vi "OceanOptics_TriggerPlayground.vi"() -> ()   [LabVIEW 2016]
uses:
  Maya2000 Typedefs/Maya2000 basic info.ctl
  <vilib>/Platform/TimedLoop/XDataNode/timing_clust.ctl
  <vilib>/Platform/TimedLoop/XDataNode/nitl_modes.ctl
  <vilib>/Platform/TimedLoop/XDataNode/wakeup.ctl
  C:/Program Files/Ocean Optics/OmniDriver/OOI_HOME/NETOmniDriver-NET40.dll
  Program Files/Ocean Optics/OmniDriver/OOI_HOME/NETOmniDriver-NET40.dll
  <vilib>/platform/TimedLoop/XDataNode/XDataNode.xnode
  <vilib>/Platform/TimedLoop/XDataNode/XDNodeRunTimeDep.lvlib
panel:
  out "getBufferCapacity 3":i32
  out "isEnableBuffer 2":i16
  out "getExternalTriggerDelayIncrement":i32
  out "read":bool
  out "getBufferCapacity":i32
  out "getNumberOfElements":i32
  out "status":bool
  out "error out":errorcluster
  out "this maya":T1={"This instruments index"=0, "Name+SerialNumber"="MayaPro2000:MAYP111403", "Number Dark pixels"=8, "NumberOfPixels\nper spectrum"=2068, "NumberOf Maya2000 instrm."=2, "MaximumIntegrationTime\n[us]"=1600000000, "MinimumIntegrationTime\n[us]"=7200}
  in  "number of scans to average":i32=1 min=1 step=1
  out "spectrum":cluster{"Y":dbl[], "Y":dbl[]}[](graph)
  in  "stop":bool
  in  "integration time [us]":i32=100000
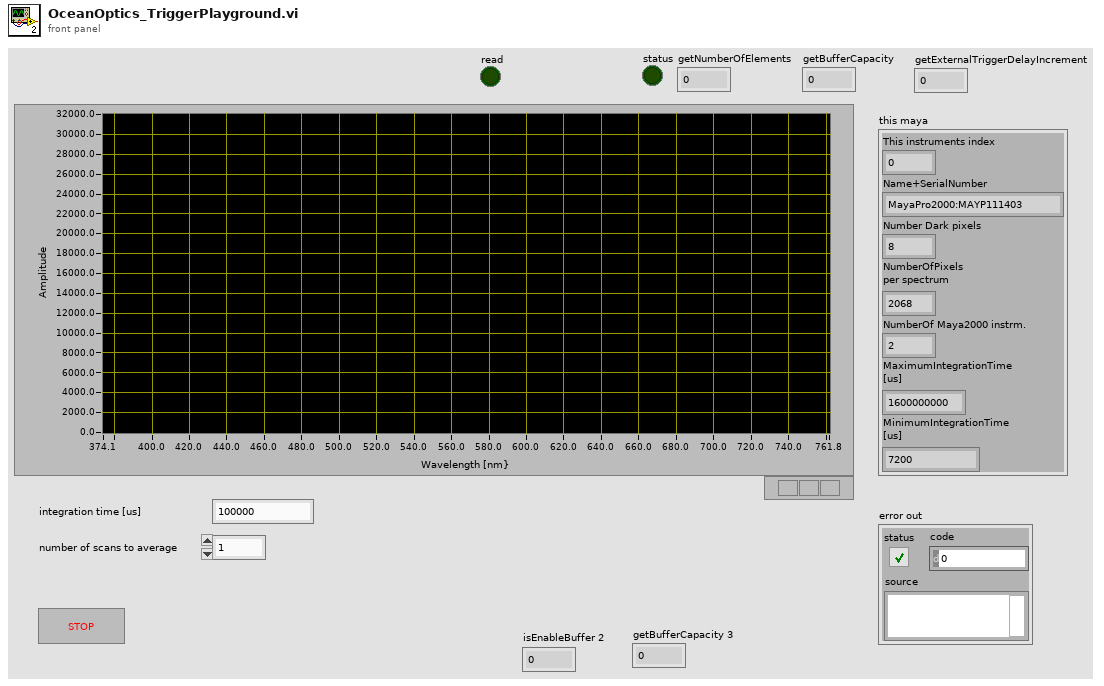
[diagram p1: front panel]
types:
  T1 = typedef "Maya2000 basic info.ctl" = cluster{"This instruments index":i32, "Name+SerialNumber":string, "Number Dark pixels":i32, "NumberOfPixels\nper spectrum":i32, "NumberOf Maya2000 instrm.":i32, "MaximumIntegrationTime\n[us]":i32, "MinimumIntegrationTime\n[us]":i32}
  T2 = typedef "XDNodeRunTimeDep.lvlib/timing_clust.ctl" = cluster{"Expected End [f-1]":u64, "Actual End [f-1]":u64, "Finished Late? [f-1]":bool, "Expected End [i-1]":u64, "Actual End [i-1]":u64, "Finished Late? [i-1]":bool, "Expected Start [i]":u64, "Actual Start [i]":u64, "Expected Start [f]":u64, "Actual Start [f]":u64, "Source Name":string, "Structure Name":string, "Period":i64, "Deadline":i64, "Offset":i64, "Start":i64, "Priority":i32, "Timeout":i32, "Mode":T3, "Wakeup Reason":T4, "Error":errorcluster, "Source Type":string, "Secondary Source Type":string, "Global End Time":u64, "Global Start Time":u64, "Frame Duration":u64, "Iteration Duration":u64, "Assigned CPU":i32, "I/O Scan Engine Mode":u32}
  T3 = typedef "XDNodeRunTimeDep.lvlib/nitl_modes.ctl" = enum32{"No Change", "Process missed periods, maintain original phase", "Discard missed periods, maintain original phase", "Process missed periods, ignore original phase", "Discard missed periods, ignore original phase"}
  T4 = typedef "XDNodeRunTimeDep.lvlib/wakeup.ctl" = enum32{"Normal", "Aborted", "Asynchronous wakeup", "Timing source error", "Timed loop error", "Timeout"}
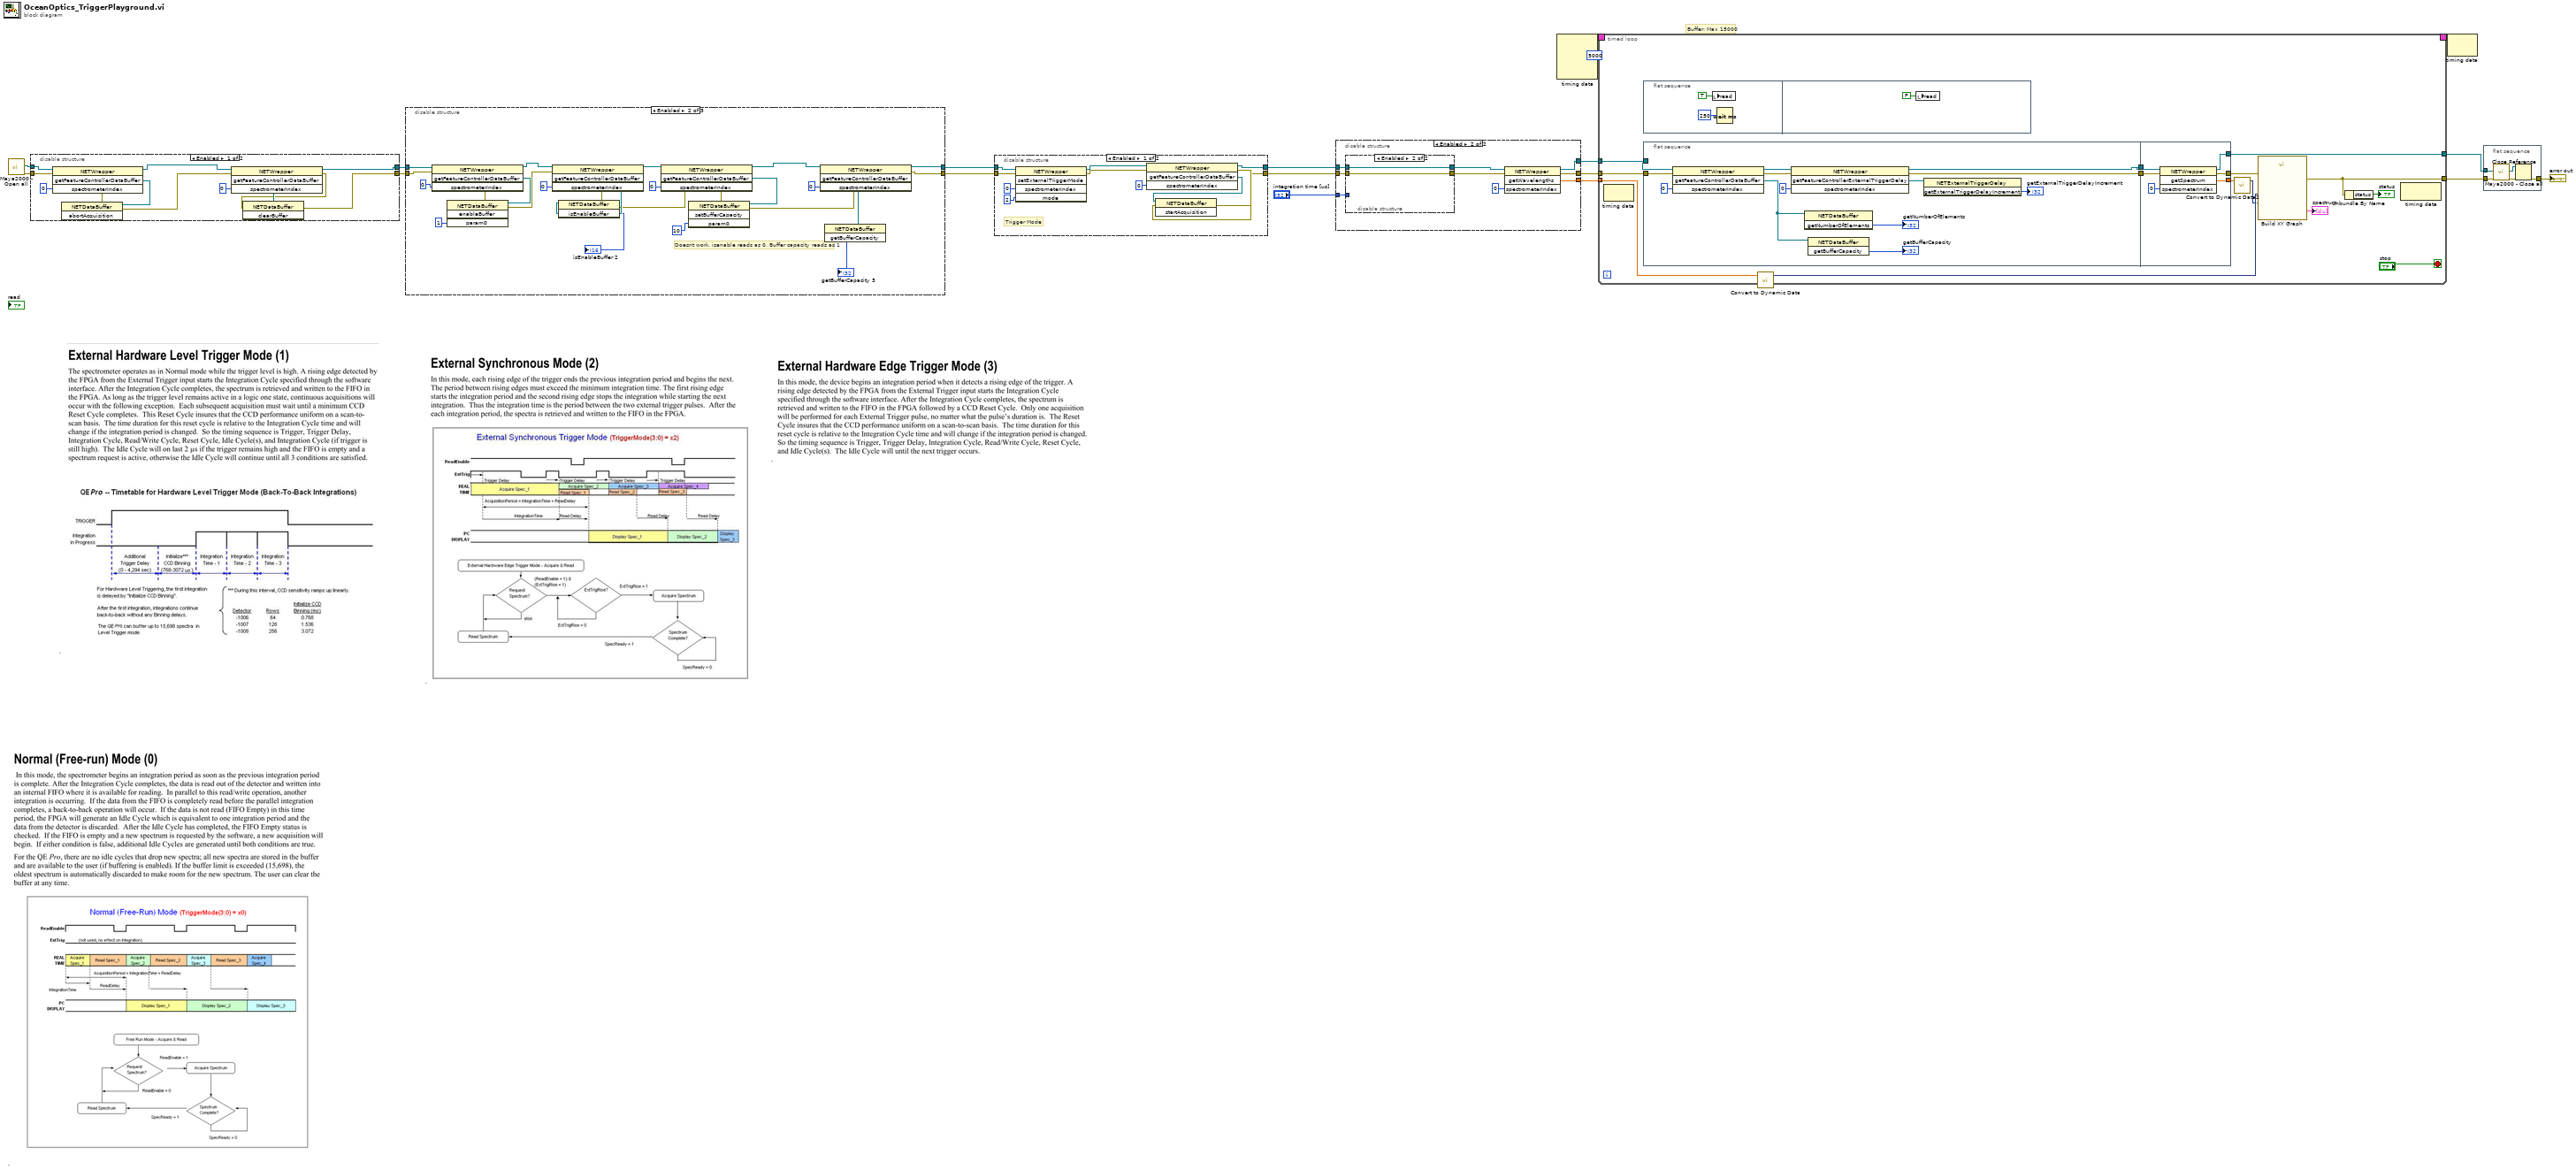
[diagram p0: block diagram]
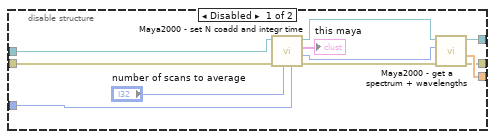
[diagram p6: hidden frame]
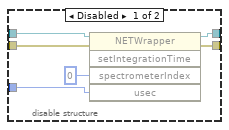
[diagram p7: hidden frame]
diagram:
  # "Buffer: Max 15000"
  n1 = call "Maya2000 - Open all.vi"() -> ("error out"=w14:errorcluster, ".NET Refnum out"=w13:refnum<k24>)  [unwired: 9 in, 1 out]
  n2 = disable-structure shown="Enabled" {
    disable-tunnel: w14 -> [w30 w31]
    disable-tunnel: w13 -> [w29 w32]
    disable-tunnel: [w19 _] -> w6
    disable-tunnel: [w21 _] -> w5
    frame Enabled {
      n3 = invoke class="NETWrapper" method="getFeatureControllerDataBuffer"(reference=w29, error in=w30, "spectrometerIndex"=0) -> (reference out=w25:refnum<k24>, error out=w27:errorcluster, "getFeatureControllerDataBuffer"=w28:refnum<k24>)  [unwired: 1 in, 1 out]
      n4 = invoke class="NETDataBuffer" method="abortAcquisition"(reference=w28, error in=w27) -> (error out=w22:errorcluster)  [unwired: 1 in, 2 out]
      n5 = invoke class="NETWrapper" method="getFeatureControllerDataBuffer"(reference=w25, error in=w22, "spectrometerIndex"=0) -> (reference out=w21:refnum<k24>, error out=w20:errorcluster, "getFeatureControllerDataBuffer"=w23:refnum<k24>)  [unwired: 1 in, 1 out]
      n6 = invoke class="NETDataBuffer" method="clearBuffer"(reference=w23, error in=w20) -> (error out=w19:errorcluster)  [unwired: 1 in, 2 out]
    }
    frame Disabled {
    }
  }
  n7 = disable-structure shown="Enabled" {
    disable-tunnel: w6 -> [_ w41 _]
    disable-tunnel: w5 -> [_ w42 _]
    disable-tunnel: [_ w46 _] -> w4
    disable-tunnel: [_ w45 _] -> w3
    frame Disabled {
    }
    frame Enabled {
      # "Doesnt work, isenable reads as 0, Buffer capacity reads as 1"
      n8 = invoke class="NETWrapper" method="getFeatureControllerDataBuffer"(reference=w42, error in=w41, "spectrometerIndex"=0) -> (reference out=w43:refnum<k24>, error out=w40:errorcluster, "getFeatureControllerDataBuffer"=w39:refnum<k24>)  [unwired: 1 in, 1 out]
      n9 = invoke class="NETDataBuffer" method="enableBuffer"(reference=w39, error in=w40, "param0"=i16 1) -> (error out=w38:errorcluster)  [unwired: 1 in, 3 out]
      n10 = invoke class="NETWrapper" method="getFeatureControllerDataBuffer"(reference=w43, error in=w38, "spectrometerIndex"=0) -> (reference out=w49:refnum<k24>, error out=w37:errorcluster, "getFeatureControllerDataBuffer"=w48:refnum<k24>)  [unwired: 1 in, 1 out]
      n11 = invoke class="NETDataBuffer" method="isEnableBuffer"(reference=w48, error in=w37) -> (error out=w36:errorcluster, "isEnableBuffer"=→"isEnableBuffer 2":i16)  [unwired: 1 in, 1 out]
      n12 = invoke class="NETWrapper" method="getFeatureControllerDataBuffer"(reference=w49, error in=w36, "spectrometerIndex"=0) -> (reference out=w54:refnum<k24>, error out=w35:errorcluster, "getFeatureControllerDataBuffer"=w56:refnum<k24>)  [unwired: 1 in, 1 out]
      n13 = invoke class="NETDataBuffer" method="setBufferCapacity"(reference=w56, error in=w35, "param0"=10) -> (error out=w34:errorcluster)  [unwired: 1 in, 3 out]
      n14 = invoke class="NETWrapper" method="getFeatureControllerDataBuffer"(reference=w54, error in=w34, "spectrometerIndex"=0) -> (reference out=w46:refnum<k24>, error out=w45:errorcluster, "getFeatureControllerDataBuffer"=w55:refnum<k24>)  [unwired: 1 in, 1 out]
      n15 = invoke class="NETDataBuffer" method="getBufferCapacity"(reference=w55) -> ("getBufferCapacity"=→"getBufferCapacity 3":i32)  [unwired: 2 in, 2 out]
    }
    frame Disabled {
    }
  }
  n16 = disable-structure shown="Enabled" {
    disable-tunnel: [w58 w69] -> w1
    disable-tunnel: [w60 w70] -> w2
    disable-tunnel: w4 -> [w66 w70]
    disable-tunnel: w3 -> [w65 w69]
    frame Enabled {
      # "Trigger Mode"
      n17 = invoke class="NETWrapper" method="setExternalTriggerMode"(reference=w66, error in=w65, "spectrometerIndex"=0, "mode"=2) -> (reference out=w63:refnum<k24>, error out=w64:errorcluster)  [unwired: 1 in, 3 out]
      n18 = invoke class="NETWrapper" method="getFeatureControllerDataBuffer"(reference=w63, error in=w64, "spectrometerIndex"=0) -> (reference out=w60:refnum<k24>, error out=w59:errorcluster, "getFeatureControllerDataBuffer"=w61:refnum<k24>)  [unwired: 1 in, 1 out]
      n19 = invoke class="NETDataBuffer" method="startAcquisition"(reference=w61, error in=w59) -> (error out=w58:errorcluster)  [unwired: 1 in, 2 out]
    }
    frame Disabled {
    }
  }
  n20 = disable-structure shown="Enabled" {
    disable-tunnel: w2 -> [w81 w88]
    disable-tunnel: w1 -> [w79 w83]
    disable-tunnel: [w75 w91] -> w15
    disable-tunnel: [w74 w86] -> w11
    disable-tunnel: [w72 w85] -> w12
    disable-tunnel: "integration time [us]" -> [w71 w87]
    frame Disabled {
      n21 = call "Maya2000 - set N coadd and integr time.vi"("Intgration time\n[us]"=w71, "numberOfScans\nToAverage"="number of scans to average", "error in (no error)"=w79, ".NET Refnum in"=w81) -> ("error out"=w76:errorcluster, "This instruments index"=w73:i32, "This Maya´\nbasic info"=→"this maya":T1, ".NET Refnum out"=w77:refnum<k24>, "Maya2000 basic values"=w80:T1[])  [unwired: 3 in]
      n22 = call "Maya2000 - get a spectrum + wavelengths.vi"("error in (no error)"=w76, "This instrments index"=w73, ".NET Refnum in"=w77) -> ("error out"=w72:errorcluster, "Wavelengths"=w75:dbl[], ".NET Refnum out"=w74:refnum<k24>)  [unwired: 3 in, 3 out]
    }
    frame Enabled {
      n23 = disable-structure shown="Enabled" {
        disable-tunnel: [w96 w98] -> w89
        disable-tunnel: w88 -> [w95 w98]
        disable-tunnel: w87 -> [w94 _]
        disable-tunnel: [w93 w99] -> w84
        disable-tunnel: w83 -> [w92 w99]
        frame Disabled {
          n24 = invoke class="NETWrapper" method="setIntegrationTime"(reference=w95, error in=w92, "spectrometerIndex"=0 ("mode"), "usec"=w94) -> (reference out=w96:refnum<k24>, error out=w93:errorcluster)  [unwired: 1 in, 3 out]
        }
        frame Enabled {
        }
      }
      n25 = invoke class="NETWrapper" method="getWavelengths"(reference=w89, error in=w84, "spectrometerIndex"=0 ("mode")) -> (reference out=w86:refnum<k24>, error out=w85:errorcluster, "getWavelengths"=w91:dbl[])  [unwired: 1 in, 1 out]
    }
  }
  n26 = node-c288(i64 5000 ("Period")) -> (w9:T2)  [unwired: 3 in]
  n27 = timed-loop {
    tunnel: [w109] -> w17
    tunnel: [w102] -> w18
    tunnel: w15 -> [w108]
    tunnel: w11 -> [w105]
    tunnel: w12 -> [w106]
    timing: w9 -> [_]
    timing-out: [_] -> w8
    stop <- "stop" stop-if-true
    n28 = node-c288() -> ()  [unwired: 1 in, 1 out]
    n29 = flat-sequence {
      frame #0 {
        n30 = local write "read"(TRUE ("read")) -> ()
        n31 = Wait (ms)(milliseconds to wait=u32 250) -> ()  [unwired: 1 out]
      }
      frame #1 {
        n32 = local write "read"(FALSE ("read")) -> ()
      }
    }
    n33 = flat-sequence {
      tunnel: w105 -> [w123]
      tunnel: w106 -> [w117]
      tunnel: [w115] -> w104
      tunnel: [w114] -> w103
      tunnel: [w129] -> w102
      tunnel: [w126] -> w101
      tunnel: w104 -> [w127]
      tunnel: w103 -> [w130]
      tunnel: [w128] -> w100
      frame #0 {
        n34 = invoke class="NETWrapper" method="getFeatureControllerDataBuffer"(reference=w123, error in=w117, "spectrometerIndex"=0) -> (error out=w116:errorcluster, "getFeatureControllerDataBuffer"=w120:refnum<k24>)  [unwired: 1 in, 2 out]
        n35 = invoke class="NETWrapper" method="getFeatureControllerExternalTriggerDelay"(reference=w123, error in=w116, "spectrometerIndex"=0) -> (reference out=w114:refnum<k24>, error out=w115:errorcluster, "getFeatureControllerExternalTriggerDelay"=w124:refnum<k24>)  [unwired: 1 in, 1 out]
        n36 = invoke class="NETDataBuffer" method="getNumberOfElements"(reference=w120) -> ("getNumberOfElements"=→"getNumberOfElements":i32)  [unwired: 2 in, 2 out]
        n37 = invoke class="NETDataBuffer" method="getBufferCapacity"(reference=w120) -> ("getBufferCapacity"=→"getBufferCapacity":i32)  [unwired: 2 in, 2 out]
        n38 = invoke class="NETExternalTriggerDelay" method="getExternalTriggerDelayIncrement"(reference=w124) -> ("getExternalTriggerDelayIncrement"=→"getExternalTriggerDelayIncrement":i32)  [unwired: 2 in, 2 out]
      }
      frame #1 {
        n39 = invoke class="NETWrapper" method="getSpectrum"(reference=w130, error in=w127, "spectrometerIndex"=0) -> (reference out=w129:refnum<k24>, error out=w126:errorcluster, "getSpectrum"=w128:dbl[])  [unwired: 1 in, 1 out]
      }
    }
    n40 = call "Convert to Dynamic Data"("Array"=w108) -> ("Dynamic Data Type"=w112:dynamicdata)  [unwired: 3 in]
    n41 = call "Convert to Dynamic Data2"("Array"=w100) -> ("Dynamic Data Type"=w111:dynamicdata)  [unwired: 3 in]
    n42 = call "Build XY Graph"("error in (no error)"=w101, "Y Input"=w111, "X Input"=w112) -> ("error out"=w109:errorcluster, "XY Graph"=→"spectrum":cluster{"X":dbl[], "Y":dbl[]}[])  [unwired: 7 in]
    n43 = Unbundle By Name(w109) -> ("status"=→"status":bool)
    n44 = node-c288() -> ()  [unwired: 1 in, 1 out]
  }
  n45 = node-c288(w8) -> ()  [unwired: 1 out]
  n46 = flat-sequence {
    tunnel: w18 -> [w141]
    tunnel: w17 -> [w140]
    tunnel: [w139] -> w16
    frame #0 {
      n47 = call "Maya2000 - Close all.vi"("error in (no error)"=w140, "Maya reference in"=w141) -> ("error out"=w138:errorcluster, ".NET Refnum out"=w137:refnum<k24>)  [unwired: 8 in]
      n48 = Close Reference(reference=w137, error in (no error)=w138) -> (error out=w139:errorcluster)
    }
  }
  "error out" <- w16
